vi "IntakeAndMagazineOutput.vi"   [LabVIEW 2019]
uses:
  <vilib>/Rock Robotics/WPI/Solenoid/WPI_SolenoidValue.ctl
  59b9c10d-8ae0-4ded-82a0-414eda02ae48.vi
  d350f25d-9219-42bc-bd22-1190862098c8.vi
  312f5e35-0350-4313-9871-8e27e988903d.vi
  ee26b6c7-8c8f-4a43-86f1-292fbd430e5b.vi
  refnums.vi
  GRNF_GenericMotor.vi
  GRNF_CTREMotor.vi
  GRNF_GenericSolenoid.vi
  outputs.vi
  dsdata.vi
  <vilib>/Rock Robotics/WPI/Solenoid/WPI_SolenoidSetEnum.vi
  TAI_Motor.vi
  TAI_Solenoid.vi
types:
  T1 = typedef "WPI_MotorControlDeviceRef.ctl" = cluster{"DeviceStatus":errorcluster, "Type":T2, "PWM":cluster{"PWM Channel":T3, "DeadBand":T4}, "CAN":cluster{"Device Number":u8, "SetOutput VI Ref":variant, "GetOutput VI Ref":variant, "Enable VI Ref":variant, "Disable VI Ref":variant, "Data":variant}, "Invert":bool, "DIO PWM":cluster{"PWM \"Enable\" Channel":T3, "DIOChannel":T5, "PWM Rate":dbl}}
  T2 = typedef "WPI_MotorControlType.ctl" = enum16{"PWM", "CAN", "DIO PWM"}
  T3 = typedef "FPGA_DIOPWMChannel.ctl" = enum8{"PWM 0", "PWM 1", "PWM 2", "PWM 3", "PWM 4", "PWM 5", "PWM 6", "PWM 7", "PWM 8", "PWM 9", "PWM MXP 0", "PWM MXP 1", "PWM MXP 2", "PWM MXP 3", "PWM MXP 4", "PWM MXP 5", "PWM MXP 6", "PWM MXP 7", "PWM MXP 8", "PWM MXP 9", "Invalid"}
  T4 = typedef "WPI_PWMDeadband.ctl" = cluster{"Name":string, "maxPositivePwm":i32, "minPositivePwm":i32, "centerPwm":i32, "maxNegativePwm":i32, "minNegativePwm":i32, "angularRange":u16}
  T5 = typedef "FPGA_DIOChannel.ctl" = enum8{"DIO 0", "DIO 1", "DIO 2", "DIO 3", "DIO 4", "DIO 5", "DIO 6", "DIO 7", "DIO 8", "DIO 9", "DIO MXP 0", "DIO MXP 1", "DIO MXP 2", "DIO MXP 3", "DIO MXP 4", "DIO MXP 5", "DIO MXP 6", "DIO MXP 7", "DIO MXP 8", "DIO MXP 9", "DIO MXP 10", "DIO MXP 11", "DIO MXP 12", "DIO MXP 13", "DIO MXP 14", "DIO MXP 15", "SPI Port CS1", "SPI Port CS2", "SPI Port CS3", "SPI Port MISO", "SPI Port MOSI", "Invalid"}
  T6 = typedef "WPI_SolenoidDevRef.ctl" = cluster{"DevStatus":errorcluster, "Pneumatics Control Module":u8, "Forward Solenoid Channel":T7, "Reverse Solenoid Channel":T7}
  T7 = typedef "WPI_SolenoidChannel.ctl" = enum8{"Solenoid 0", "Solenoid 1", "Solenoid 2", "Solenoid 3", "Solenoid 4", "Solenoid 5", "Solenoid 6", "Solenoid 7", "Invalid"}
  T8 = typedef "WPI_DriverStationRobotMode2.ctl" = enum16{"Autonomous Disabled", "Autonomous Enabled", "Teleop Disabled", "Teleop Enabled", "Disconnected", "Finish", "Test Disabled", "Test Enabled", "Emergency Stopped"}
  T9 = typedef "WPI_SolenoidValue.ctl" = enum16{"Off", "On", "Forward", "Reverse"}
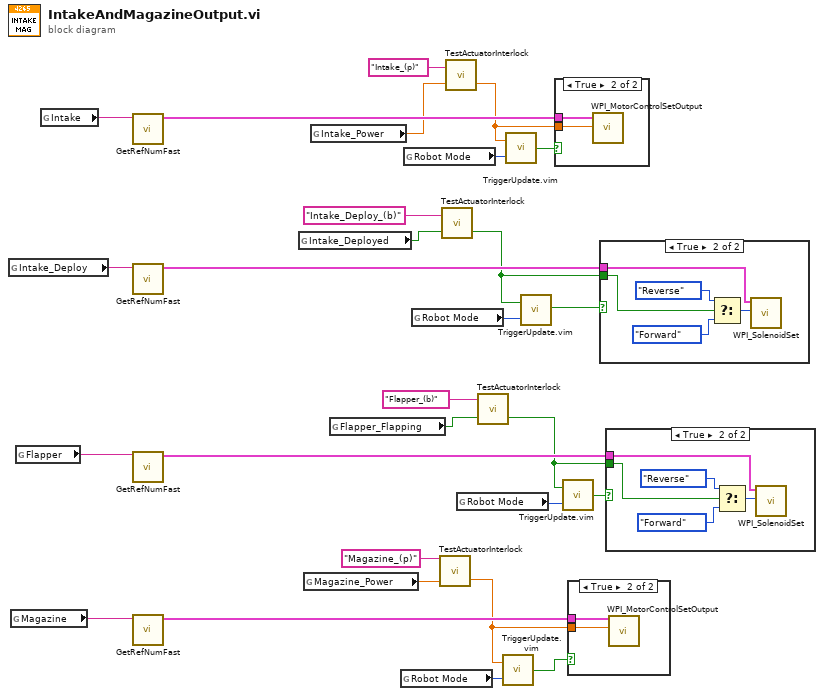
[diagram p0: block diagram]
diagram:
  n1 = global read "refnums.vi" "Intake_Deploy"() -> (w15:string)
  n2 = global read "refnums.vi" "Magazine"() -> (w13:string)
  n3 = global read "refnums.vi" "Flapper"() -> (w14:string)
  n4 = global read "refnums.vi" "Intake"() -> (w16:string)
  n5 = call-poly "GetRefNumFast.vi"("RefNum Name"=w16) -> ("Device Reference"=w20:T1)  [unwired: 5 in, 1 out]
  n6 = call-poly "GetRefNumFast.vi"("RefNum Name"=w15) -> ("Device Reference"=w19:T6)  [unwired: 5 in, 1 out]
  n7 = call-poly "GetRefNumFast.vi"("RefNum Name"=w14) -> ("Device Reference"=w18:T6)  [unwired: 5 in, 1 out]
  n8 = call-poly "GetRefNumFast.vi"("RefNum Name"=w13) -> ("Device Reference"=w17:T1)  [unwired: 5 in, 1 out]
  n9 = global read "outputs.vi" "Intake_Deployed"() -> (w8:bool)
  n10 = global read "outputs.vi" "Magazine_Power"() -> (w1:dbl)
  n11 = global read "outputs.vi" "Intake_Power"() -> (w10:dbl)
  n12 = global read "outputs.vi" "Flapper_Flapping"() -> (w4:bool)
  n13 = global read "dsdata.vi" "Robot Mode"() -> (w23:T8)
  n14 = global read "dsdata.vi" "Robot Mode"() -> (w22:T8)
  n15 = global read "dsdata.vi" "Robot Mode"() -> (w24:T8)
  n16 = call-poly "TestActuatorInterlock.vi"("Normal Output"=w1, "Actuator Name"="Magazine_(p)" ("Actuator_Name")) -> ("Interlock Output"=w3:dbl)  [unwired: 1 out]
  n17 = call-poly "TestActuatorInterlock.vi"("Normal Output"=w8, "Actuator Name"="Intake_Deploy_(b)" ("Actuator_Name")) -> ("Interlock Output"=w9:bool)  [unwired: 1 out]
  n18 = call-poly "TestActuatorInterlock.vi"("Normal Output"=w10, "Actuator Name"="Intake_(p)" ("Actuator_Name")) -> ("Interlock Output"=w12:dbl)  [unwired: 1 out]
  n19 = global read "dsdata.vi" "Robot Mode"() -> (w26:T8)
  n20 = call-poly "TestActuatorInterlock.vi"("Normal Output"=w4, "Actuator Name"="Flapper_(b)" ("Actuator_Name")) -> ("Interlock Output"=w6:bool)  [unwired: 1 out]
  n21 = call "TriggerUpdate.vim"("Robot Mode"=w23, "Trigger"=w3) -> ("Update"=w28:bool)
  n22 = call "TriggerUpdate.vim"("Robot Mode"=w22, "Trigger"=w12) -> ("Update"=w21:bool)
  n23 = call "TriggerUpdate.vim"("Robot Mode"=w24, "Trigger"=w9) -> ("Update"=w25:bool)
  n24 = case shown="True" w21 {
    tunnel: w20 -> [_ w30]
    tunnel: w12 -> [_ w29]
    frame False {
    }
    frame True {
      n25 = call <vilib>:"WPI_MotorControlSetOutput.vi"("Output"=w29, "MotorControlDevRef"=w30) -> ()  [unwired: 7 in, 3 out]
    }
  }
  n26 = call "TriggerUpdate.vim"("Robot Mode"=w26, "Trigger"=w6) -> ("Update"=w27:bool)
  n27 = case shown="True" w28 {
    tunnel: w17 -> [_ w32]
    tunnel: w3 -> [_ w31]
    frame False {
    }
    frame True {
      n28 = call <vilib>:"WPI_MotorControlSetOutput.vi"("Output"=w31, "MotorControlDevRef"=w32) -> ()  [unwired: 7 in, 3 out]
    }
  }
  n29 = case shown="True" w25 {
    tunnel: w9 -> [_ w33]
    tunnel: w19 -> [_ w34]
    frame False {
    }
    frame True {
      n30 = Select(t=WPI_SolenoidValue."Reverse" ("Value"), s=w33, f=WPI_SolenoidValue."Forward" ("Value")) -> (s? t:f=w37:T9)
      n31 = call-poly <vilib>:"WPI_SolenoidSet.vi"("Value"=w37, "SolenoidDevRef"=w34) -> ()  [unwired: 8 in, 2 out]
    }
  }
  n32 = case shown="True" w27 {
    tunnel: w6 -> [_ w38]
    tunnel: w18 -> [_ w39]
    frame False {
    }
    frame True {
      n33 = Select(t=WPI_SolenoidValue."Reverse" ("Value"), s=w38, f=WPI_SolenoidValue."Forward" ("Value")) -> (s? t:f=w42:T9)
      n34 = call-poly <vilib>:"WPI_SolenoidSet.vi"("Value"=w42, "SolenoidDevRef"=w39) -> ()  [unwired: 8 in, 2 out]
    }
  }
